vi "Read Spectrum.vi"(0 "VISA Session":refnum<visa-resource-name>="GPIB1::9::INSTR", 11 "Error In":errorcluster) -> (4 "Copy VISA Session":refnum<visa-resource-name>, 6 "Wavelike Data (X)":dbl[](array[numeric]) format="%.12f", 8 "Wavelike Data (Y)":dbl[](array[numeric]) format="%.12f", 15 "Error Out":errorcluster)   [LabVIEW 2021]
panel:
  # "Antes de utilizar esta VI, deve-se executar a VI de configuração \ndo espectrômetro (Config Spectrometer.vi)."
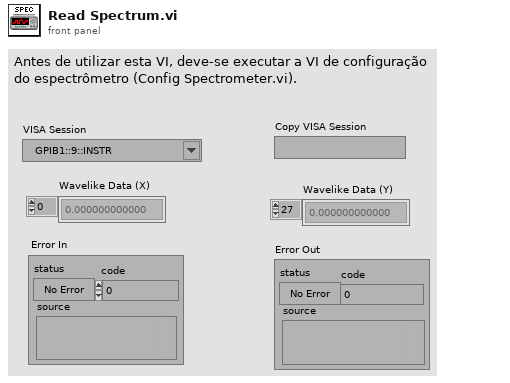
[diagram p1: front panel]
types:
  T1 = enum16{"Y AXIS Data Output", "X AXIS Data Output"}
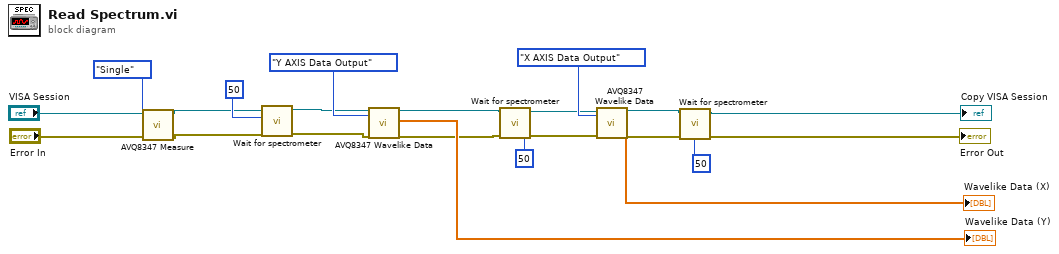
[diagram p0: block diagram]
diagram:
  n1 = call "AVQ8347 Measure.vi"("Error In"="Error In", "Measure Select"=enum16{"Stop", "Single", "Repeat"}."Single", "VISA Session"="VISA Session") -> ("Error Out"=w5:errorcluster, "Copy VISA Session"=w6:refnum<visa-resource-name>)  [unwired: 6 in, 1 out]
  n2 = call "Wait for spectrometer.vi"("error in (no error)"=w5, "milliseconds to wait"=u32 50, "VISA Refnum in"=w6) -> ("error out"=w15:errorcluster, "VISA Refnum out"=w16:refnum<visa-resource-name>)  [unwired: 6 in, 1 out]
  n3 = call "AVQ8347 Wavelike Data.vi"("VISA Session"=w16, "Axis Select"=T1."Y AXIS Data Output", "Error In"=w15) -> ("Copy VISA Session"=w9:refnum<visa-resource-name>, "Wavelike Data"=→"Wavelike Data (Y)":dbl[], "Error Out"=w11:errorcluster)  [unwired: 12 in, 2 out]
  n4 = call "Wait for spectrometer.vi"("error in (no error)"=w11, "milliseconds to wait"=u32 50, "VISA Refnum in"=w9) -> ("error out"=w12:errorcluster, "VISA Refnum out"=w13:refnum<visa-resource-name>)  [unwired: 6 in, 1 out]
  n5 = call "AVQ8347 Wavelike Data.vi"("VISA Session"=w13, "Axis Select"=T1."X AXIS Data Output", "Error In"=w12) -> ("Copy VISA Session"=w8:refnum<visa-resource-name>, "Wavelike Data"=→"Wavelike Data (X)":dbl[], "Error Out"=w10:errorcluster)  [unwired: 12 in, 2 out]
  n6 = call "Wait for spectrometer.vi"("error in (no error)"=w10, "milliseconds to wait"=u32 50, "VISA Refnum in"=w8) -> ("error out"=→"Error Out":errorcluster, "VISA Refnum out"=→"Copy VISA Session":refnum<visa-resource-name>)  [unwired: 6 in, 1 out]
